vi "FGV User Event Reference Manager.vi"(7 "Method (Get User Event Ref)":T2=enum."Get User Event Ref", 8 "error in (no error)":errorcluster, 11 "User Event Name":string) -> (0 "error out":errorcluster, 1 "Valid Data Set?":bool, 2 "User Event Ref  Out":T1, 3 "All User Event Refs Out":T1[](array[typedef]))   [LabVIEW 2009]
doc: "This is a copy of the solution to the functional global variable exercise. It manages User Events in the Wind Farm example.\n\nAAL 9/09"
uses:
  Controls/TYPE FGV User Event Method.ctl
  Controls/TYPE FGV User Event Ref.ctl
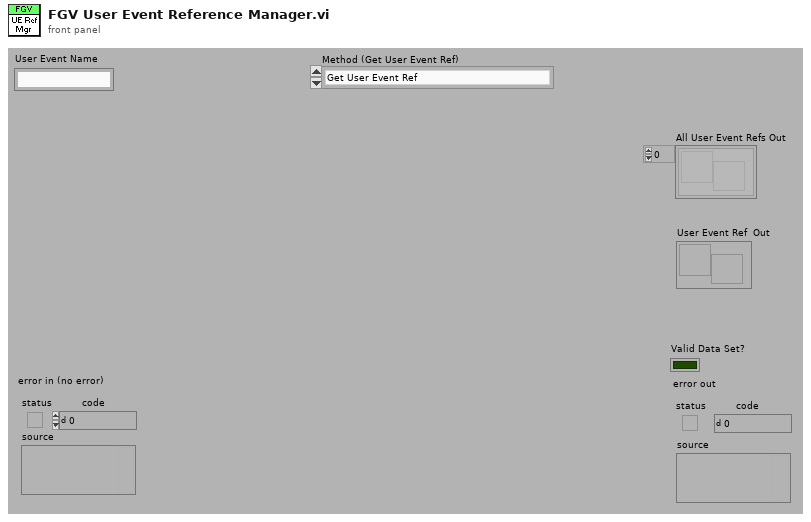
[diagram p1: front panel]
types:
  T1 = typedef "TYPE FGV User Event Ref.ctl" = refnum<user-event>
  T2 = typedef "TYPE FGV User Event Method.ctl" = enum16{"Add User Event Ref", "Modify User Event Ref", "Get User Event Ref", "Delete User Event Ref", "Get All User Event Refs", "Delete All User Event Refs"}
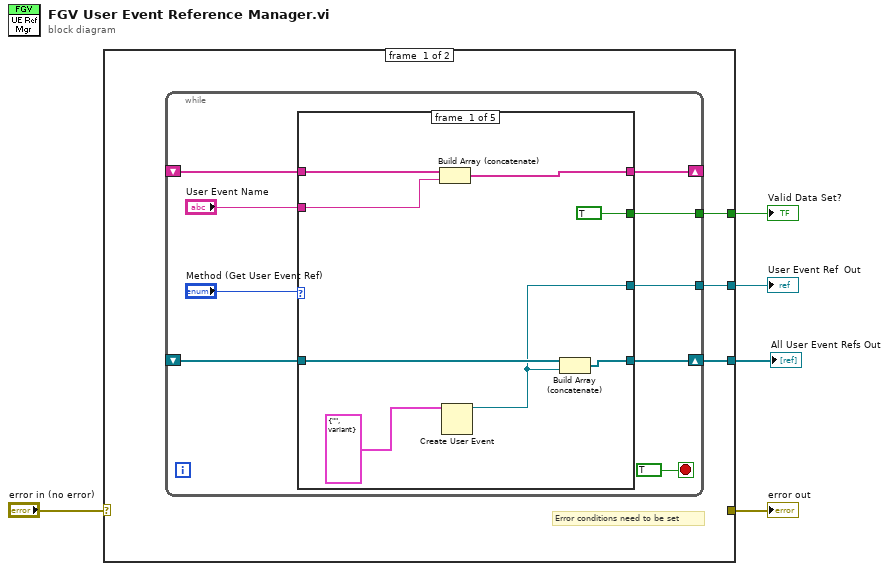
[diagram p0: block diagram]
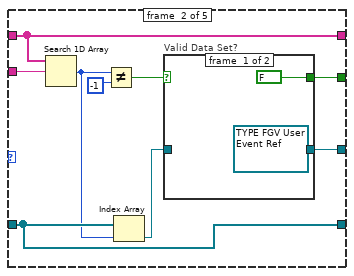
[diagram p2: hidden frame]
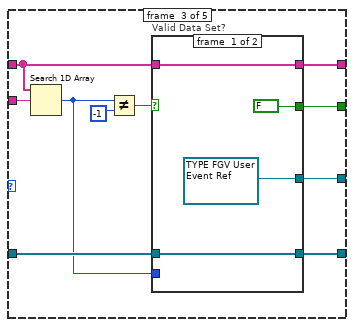
[diagram p4: hidden frame]
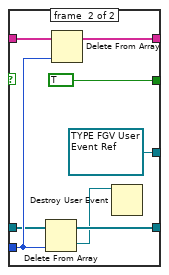
[diagram p5: hidden frame]
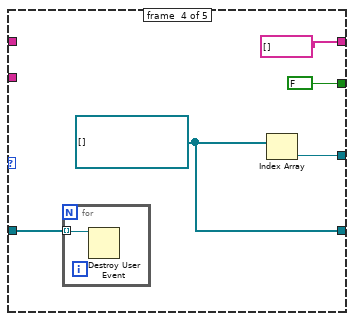
[diagram p6: hidden frame]
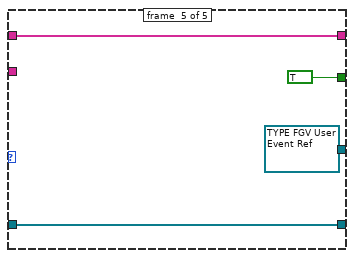
[diagram p7: hidden frame]
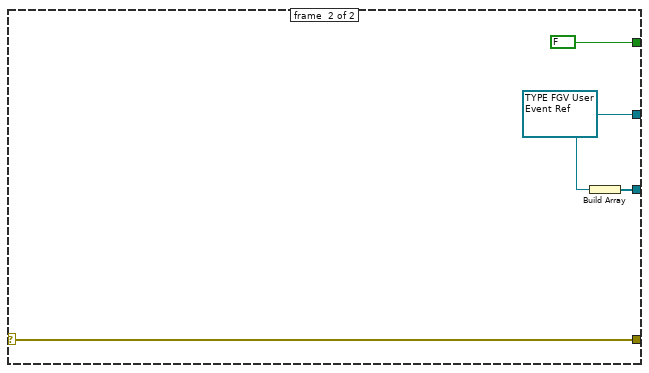
[diagram p8: hidden frame]
diagram:
  n1 = case shown="No Error" "error in (no error)" {
    selector: "error in (no error)" -> [_ w74]
    tunnel: [_ w74] -> w4
    tunnel: [w8 w72] -> w3
    tunnel: [w7 FALSE] -> w2
    tunnel: [w6 w71] -> w1
    frame #0 {
      # "Error conditions need to be set"
      n2 = while {
        shift-right: [w14] -> _
        shift-left: _ -> [w13]
        shift-right: [w9] -> w6
        shift-left: _ -> [w11]
        tunnel: [w12] -> w8
        tunnel: [w10] -> w7
        stop <- TRUE stop-if-true
        n3 = case shown="\"Add User Event Ref\"" "Method (Get User Event Ref)" {
          tunnel: "User Event Name" -> [w19 w34 w48 _ _]
          tunnel: [w25 w33 w47 string[] [] w70] -> w14
          tunnel: w13 -> [w24 w33 w39 _ w70]
          tunnel: [w18 w32 w45 w63 w68] -> w9
          tunnel: w11 -> [w23 w32 w46 w61 w68]
          tunnel: [w20 w27 w40 w62 T1 refnum ("Loop Data")] -> w12
          tunnel: [TRUE w28 w44 FALSE TRUE] -> w10
          frame #0 {
            n4 = Build Array (concatenate)(w24, w19) -> (w25:string[])
            n5 = Create User Event(user event datatype=cluster{"String":string, "Data":variant} {"String"="", "Data"=variant} ("User Event")) -> (user event=w20:refnum<user-event>)  [unwired: 1 in, 1 out]
            n6 = Build Array (concatenate)(w23, w20) -> (w18:T1[])
          }
          frame #1 {
            n7 = Search 1D Array(1D array=w33, element=w34) -> (index of element=w30:i32)  [unwired: 1 out]
            n8 = Not Equal?(x=w30, y=-1 ("index of element")) -> (x != y?=w31:bool)
            n9 = Index Array(array=w32, index=w30) -> (element=w26:T1)
            n10 = case "Valid Data Set?" shown="False" w31 {
              selector: w31 -> [_ w38]
              tunnel: [FALSE w38] -> w28
              tunnel: [T1 refnum ("DataSet Data") w37] -> w27
              tunnel: w26 -> [_ w37]
              frame #0 {
              }
              frame #1 {
              }
            }
          }
          frame #2 {
            n11 = Search 1D Array(1D array=w39, element=w48) -> (index of element=w42:i32)  [unwired: 1 out]
            n12 = Not Equal?(x=w42, y=-1 ("index of element")) -> (x != y?=w41:bool)
            n13 = case "Valid Data Set?" shown="True" w41 {
              tunnel: w39 -> [w52 w55]
              tunnel: w42 -> [_ w60]
              tunnel: [w52 w59] -> w47
              tunnel: w46 -> [w50 w58]
              tunnel: [w50 w57] -> w45
              tunnel: [FALSE TRUE] -> w44
              tunnel: [T1 refnum ("Loop Data") T1 refnum ("Loop Data")] -> w40
              frame #0 {
              }
              frame #1 {
                n14 = Delete From Array(array=w58, index=w60) -> (deleted portion=w54:T1, array with subset deleted=w57:T1[])  [unwired: 1 in]
                n15 = Delete From Array(array=w55, index=w60) -> (array with subset deleted=w59:string[])  [unwired: 1 in, 1 out]
                n16 = Destroy User Event(user event=w54) -> ()  [unwired: 1 in, 1 out]
              }
            }
          }
          frame #3 {
            w63 = T1[] []
            n17 = for {
              tunnel: w61 -> [w66] mode=indexing
              n18 = Destroy User Event(user event=w66) -> ()  [unwired: 1 in, 1 out]
            }
            n19 = Index Array(array=w63) -> (element=w62:T1)  [unwired: 1 in]
          }
          frame #4 {
          }
        }
      }
    }
    frame #1 {
      w72 = T1 refnum ("Loop Data")
      n20 = Build Array(w72) -> (w71:T1[])
    }
  }
  "error out" <- w4
  "User Event Ref  Out" <- w3
  "Valid Data Set?" <- w2
  "All User Event Refs Out" <- w1
